vi "SaveUISettings.vi"(8 "Error In":errorcluster, 11 "UI References":T1) -> (0 "Error Out":errorcluster)   [LabVIEW 2017, in "Client.lvlib" / "UI_API.lvlib"]
uses:
  UI_API.lvlib
  NI_LVConfig.lvlib
  Client.lvlib
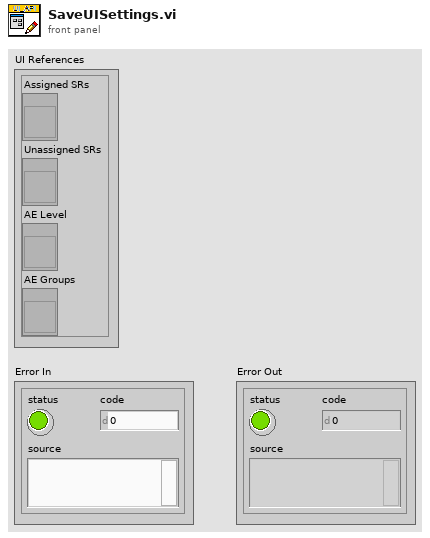
[diagram p1: front panel]
types:
  T1 = cluster{"Assigned SRs":refnum<vi>, "Unassigned SRs":refnum<vi>, "AE Level":refnum<vi>, "AE Groups":refnum<vi>}
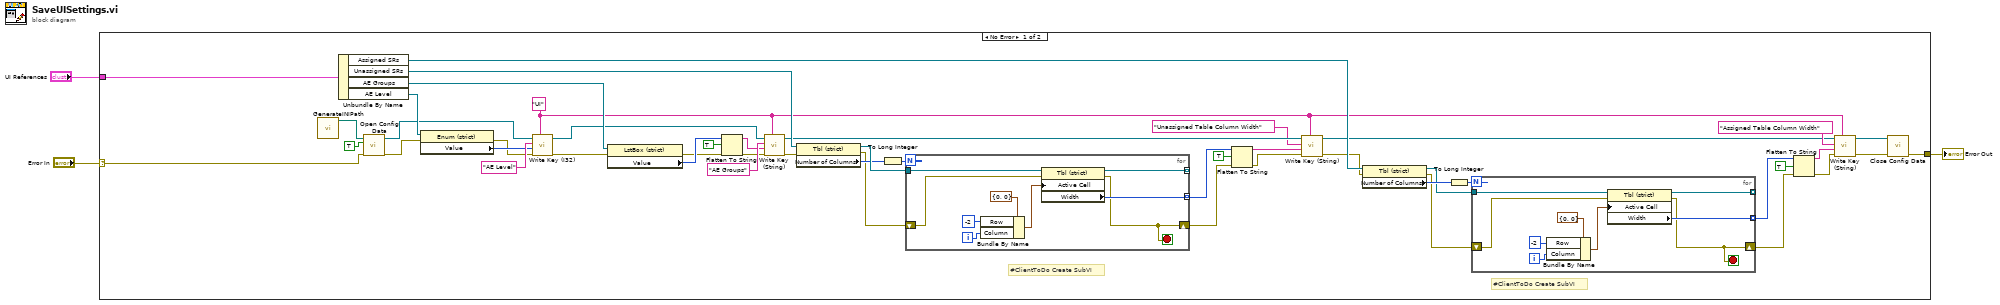
[diagram p0: block diagram]
diagram:
  n1 = case shown="No Error" "Error In" {
    selector: "Error In" -> [w51 w71]
    tunnel: "UI References" -> [w50 _]
    tunnel: [w34 w71] -> w1
    frame No Error {
      w14 = "UI" ("section")
      # "#ClientToDo Create SubVI"
      # "#ClientToDo Create SubVI"
      n2 = call "GenerateINIPath.vi"() -> ("INI Path"=w4:path)  [unwired: 11 in]
      n3 = Unbundle By Name(w50) -> ("Assigned SRs"=w20:refnum<vi>, "Unassigned SRs"=w33:refnum<vi>, "AE Groups"=w42:refnum<vi>, "AE Level"=w48:refnum<vi>)
      n4 = call "Open Config Data.vi"("error in (no error)"=w51, "create file if necessary (T)"=TRUE ("create file if necessary? (T)"), "configuration file path"=w4) -> ("error out"=w46:errorcluster, "refnum"=w44:refnum<k1>)  [unwired: 6 in, 1 out]
      n5 = property class="Enum (strict)"(reference=w48, error in=w46) -> (error out=w45:errorcluster, "Value"=w47:enum16{"AE / ELP", "AE Intern"})  [unwired: 1 out]
      n6 = call "Write Key (I32).vi"("section"=w14, "error in (no error)"=w45, "value"=w47, "key"="AE Level", "refnum"=w44) -> ("error out"=w41:errorcluster, "refnum out"=w35:refnum<k1>)  [unwired: 4 in, 1 out]
      n7 = property class="LstBox (strict)"(reference=w42, error in=w41) -> (error out=w37:errorcluster, "Value"=w40:i32[])  [unwired: 1 out]
      n8 = Flatten To String(anything=w40, prepend array or string size? (T)=TRUE, error in (no error)=w37) -> (data string=w38:string, error out=w36:errorcluster)  [unwired: 1 in, 1 out]
      n9 = call "Write Key (String).vi"("section"=w14, "error in (no error)"=w36, "value"=w38, "key"="AE Groups", "refnum"=w35) -> ("error out"=w17:errorcluster, "refnum out"=w27:refnum<k1>)  [unwired: 4 in, 1 out]
      n10 = property class="Tbl (strict)"(reference=w33, error in=w17) -> (reference out=w32:refnum<vi>, error out=w18:errorcluster, "Number of Columns"=w31:u32)
      n11 = To Long Integer(number=w31) -> (32bit integer=w30:i32)
      n12 = for {
        N: w30 -> [_]
        shift-right: [w63] -> w19
        shift-left: w18 -> [w64]
        tunnel: w32 -> [w70]
        tunnel: [w66] -> w28 mode=indexing
        tunnel: [w65] -> _ mode=indexing
        i -> [w62]
        stop <- w63 stop-if-true
        n13 = Bundle By Name(cluster=cluster{"Row":i32, "Column":i32} {"Row"=0, "Column"=0} ("Active Cell:Active Cell"), "Row"=-2, "Column"=w62) -> (w67:cluster{"Row":i32, "Column":i32})
        n14 = property class="Tbl (strict)"(reference=w70, error in=w64, "Active Cell"=w67) -> (reference out=w65:refnum<vi>, error out=w63:errorcluster, "Width"=w66:u32)
      }
      n15 = Flatten To String(anything=w28, prepend array or string size? (T)=TRUE, error in (no error)=w19) -> (data string=w25:string, error out=w26:errorcluster)  [unwired: 1 in, 1 out]
      n16 = call "Write Key (String).vi"("section"=w14, "error in (no error)"=w26, "value"=w25, "key"="Unassigned Table Column Width", "refnum"=w27) -> ("error out"=w13:errorcluster, "refnum out"=w11:refnum<k1>)  [unwired: 4 in, 1 out]
      n17 = property class="Tbl (strict)"(reference=w20, error in=w13) -> (reference out=w21:refnum<vi>, error out=w16:errorcluster, "Number of Columns"=w22:u32)
      n18 = To Long Integer(number=w22) -> (32bit integer=w23:i32)
      n19 = for {
        N: w23 -> [_]
        shift-right: [w54] -> w8
        shift-left: w16 -> [w55]
        tunnel: w21 -> [w61]
        tunnel: [w57] -> w7 mode=indexing
        tunnel: [w56] -> _ mode=indexing
        i -> [w53]
        stop <- w54 stop-if-true
        n20 = Bundle By Name(cluster=cluster{"Row":i32, "Column":i32} {"Row"=0, "Column"=0} ("Active Cell:Active Cell"), "Row"=-2, "Column"=w53) -> (w58:cluster{"Row":i32, "Column":i32})
        n21 = property class="Tbl (strict)"(reference=w61, error in=w55, "Active Cell"=w58) -> (reference out=w56:refnum<vi>, error out=w54:errorcluster, "Width"=w57:u32)
      }
      n22 = Flatten To String(anything=w7, prepend array or string size? (T)=TRUE, error in (no error)=w8) -> (data string=w5:string, error out=w6:errorcluster)  [unwired: 1 in, 1 out]
      n23 = call "Write Key (String).vi"("section"=w14, "error in (no error)"=w6, "value"=w5, "key"="Assigned Table Column Width", "refnum"=w11) -> ("error out"=w12:errorcluster, "refnum out"=w10:refnum<k1>)  [unwired: 4 in, 1 out]
      n24 = call "Close Config Data.vi"("error in (no error)"=w12, "refnum"=w10) -> ("error out"=w34:errorcluster)  [unwired: 8 in, 1 out]
    }
    frame Error {
    }
  }
  "Error Out" <- w1
